vi "svfa_Check for Window Change (Dual).vi"(4 "force/exp settings":T1={"force window [%]"=50.0, "exp window [%]"=10.0} {"exp window [%]" min=0.0 max=100.0 format="%.2f"; "force window [%]" min=0.0 max=100.0 format="%.2f"}, 6 "window":T2 items=["None"=0, "Hanning"=1, "Hamming"=2, "Blackman-Harris"=3, "Exact Blackman"=4, "Blackman"=5, "Flat Top"=6, "4 Term B-Harris "=7, "7 Term B-Harris"=8, "Low Sidelobe"=9, "Force - Exponential"=10, "Blackman Nuttall"=11, "Triangle"=30, "Bartlett-Hanning"=31, "Bohman"=32, "Parzen"=33, "Welch"=34, "Kaiser"=60, "Dolph-Chebyshev"=61, "Gaussian"=62], 7 "restart averaging (F)":bool, 8 "error in (no error)":errorcluster) -> (0 "error out":errorcluster, 1 "parameter has changed":bool)   [LabVIEW 2017]
uses:
  <vilib>/addons/_NISVFA/_Shared subVIs/Controls/svc_Window [Dual FFT].ctl
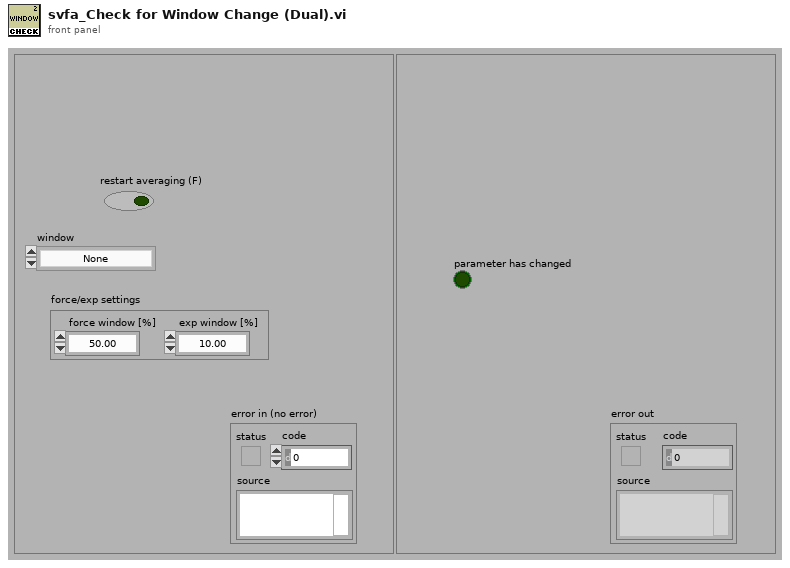
[diagram p1: front panel]
types:
  T1 = cluster{"force window [%]":dbl, "exp window [%]":dbl}
  T2 = typedef "svc_Window [Dual FFT].ctl" = u32
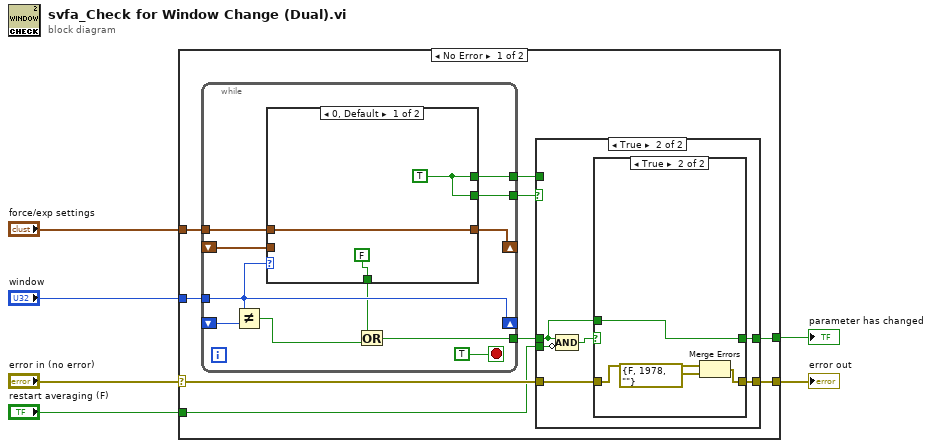
[diagram p0: block diagram]
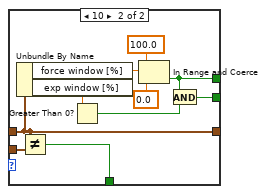
[diagram p2: hidden frame]
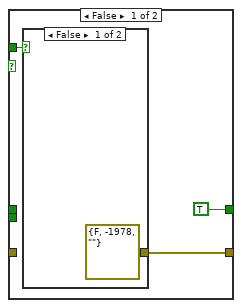
[diagram p3: hidden frame]
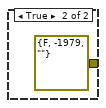
[diagram p4: hidden frame]
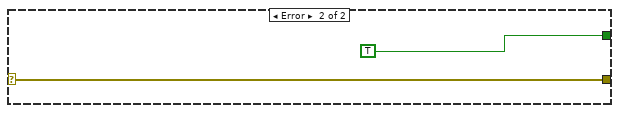
[diagram p6: hidden frame]
diagram:
  n1 = case shown="No Error" "error in (no error)" {
    selector: "error in (no error)" -> [w8 w58]
    tunnel: "window" -> [w15 _]
    tunnel: [w10 TRUE] -> w5
    tunnel: "force/exp settings" -> [w13 _]
    tunnel: [w9 w58] -> w2
    tunnel: "restart averaging (F)" -> [w7 _]
    frame No Error {
      n2 = while {
        tunnel: [w16] -> w11
        tunnel: [w17] -> w12
        tunnel: w13 -> [w23]
        shift-left: _ -> [w21]
        shift-right: [w22] -> _
        tunnel: [w18] -> w14
        tunnel: w15 -> [w24]
        shift-left: _ -> [w25]
        shift-right: [w24] -> _
        stop <- TRUE stop-if-true
        n3 = Not Equal?(x=w24, y=w25) -> (x != y?=w20:bool)
        n4 = case shown="0, Default" w24 {
          tunnel: w23 -> [w28 w33]
          tunnel: [w28 w33] -> w22
          tunnel: w21 -> [_ w34]
          tunnel: [FALSE w32] -> w19
          tunnel: [w27 w31] -> w17
          tunnel: [w27 w30] -> w16
          frame 0, Default {
            w27 = TRUE
          }
          frame 10 {
            n5 = Unbundle By Name(w33) -> ("force window [%]"=w38:dbl, "exp window [%]"=w39:dbl)
            n6 = Not Equal?(x=w33, y=w34) -> (x != y?=w32:bool)
            n7 = Greater Than 0?(x=w39) -> (x > 0?=w35:bool)
            n8 = In Range and Coerce(upper limit=100.0, x=w38, lower limit=0.0) -> (In Range?=w30:bool)  [unwired: 1 out]
            n9 = And(x=w30, y=w35) -> (x .and. y?=w31:bool)
          }
        }
        n10 = Or(x=w19, y=w20) -> (x .or. y?=w18:bool)
      }
      n11 = case shown="True" w12 {
        tunnel: w11 -> [w42 _]
        tunnel: w14 -> [_ w45]
        tunnel: [TRUE w50] -> w10
        tunnel: [w40 w49] -> w9
        tunnel: w8 -> [_ w48]
        tunnel: w7 -> [_ w47]
        frame False {
          n12 = case shown="False" w42 {
            tunnel: [errorcluster {"status"=FALSE, "code"=-1978, "source"=""} ("error IO") errorcluster {"status"=FALSE, "code"=-1979, "source"=""} ("error IO")] -> w40
            frame False {
            }
            frame True {
            }
          }
        }
        frame True {
          n13 = Compound Arithmetic op=AND(w45, invert w47) -> (w46:bool)
          n14 = case shown="True" w46 {
            tunnel: [w51 w56] -> w50
            tunnel: [w52 w53] -> w49
            tunnel: w48 -> [w52 w55]
            tunnel: w45 -> [w51 w56]
            frame False {
            }
            frame True {
              n15 = Merge Errors(w55, errorcluster {"status"=FALSE, "code"=1978, "source"=""} ("error IO")) -> (w53:errorcluster)
            }
          }
        }
      }
    }
    frame Error {
    }
  }
  "error out" <- w2
  "parameter has changed" <- w5
